vi "path to path array.vi"(8 "error in (no error)":errorcluster, 11 "path":string) -> (0 "error out":errorcluster, 3 "path array":string[](array[string]))   [LabVIEW 2016, in "JSON Value.lvclass"]
uses:
  JSON Value.lvclass
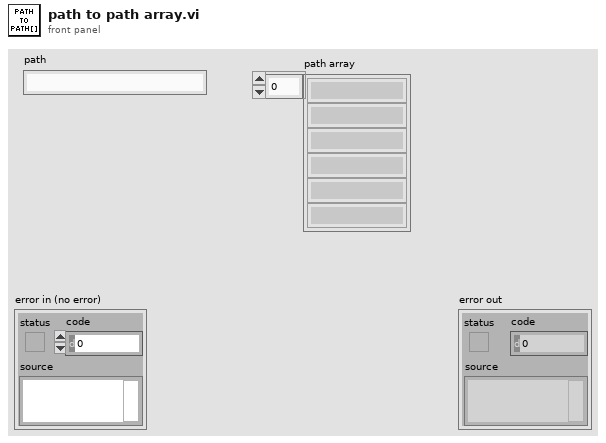
[diagram p1: front panel]
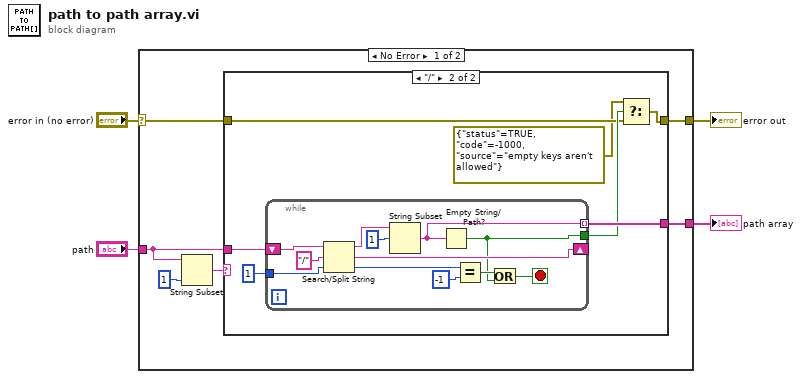
[diagram p0: block diagram]
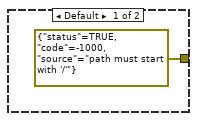
[diagram p2: hidden frame]
diagram:
  n1 = case shown="No Error" "error in (no error)" {
    selector: "error in (no error)" -> [w5 w31]
    tunnel: [w8 w31] -> w3
    tunnel: "path" -> [w7 _]
    tunnel: [w6 _] -> w1
    frame No Error {
      n2 = String Subset(string=w7, length (rest)=1 ("length (rest)")) -> (substring=w9:string)  [unwired: 1 in]
      n3 = case shown="\"/\"" w9 {
        tunnel: [errorcluster {"status"=TRUE, "code"=-1000, "source"="path must start with '/'"} ("error IO") w13] -> w8
        tunnel: w7 -> [_ w17]
        tunnel: [_ w18] -> w6
        tunnel: w5 -> [_ w14]
        frame Default {
        }
        frame "/" {
          n4 = while {
            tunnel: [w21] -> w18 mode=indexing
            shift-right: [w30] -> _
            shift-left: w17 -> [w25]
            tunnel: 1 ("length (rest)") -> [w22]
            tunnel: [w19] -> w15
            stop <- w20 stop-if-true
            n5 = Search/Split String(string=w25, search string/char (-)="/", offset (0)=w22) -> (substring before match=w23:string, match + rest of string=w30:string, offset of match=w28:i32)
            n6 = String Subset(string=w23, offset (0)=1) -> (substring=w21:string)  [unwired: 1 in]
            n7 = Empty String/Path?(string/path=w21) -> (empty?=w19:bool)
            n8 = Equal?(x=w28, y=-1) -> (x = y?=w26:bool)
            n9 = Or(x=w26, y=w19) -> (x .or. y?=w20:bool)
          }
          n10 = Select(t=errorcluster {"status"=TRUE, "code"=-1000, "source"="empty keys aren't allowed"}, s=w15, f=w14) -> (s? t:f=w13:errorcluster)
        }
      }
    }
    frame Error {
    }
  }
  "error out" <- w3
  "path array" <- w1
